vi "RestartPC ver2016 - Labview.vi"() -> ()   [LabVIEW 2016]
uses:
  System.Windows.Forms
  System.Drawing
panel:
  out "error out 3":errorcluster
  in  "error in (no error)":errorcluster
  out "error out":errorcluster
  out "standard output":string
  out "error out 2":errorcluster
  in  "stop":bool
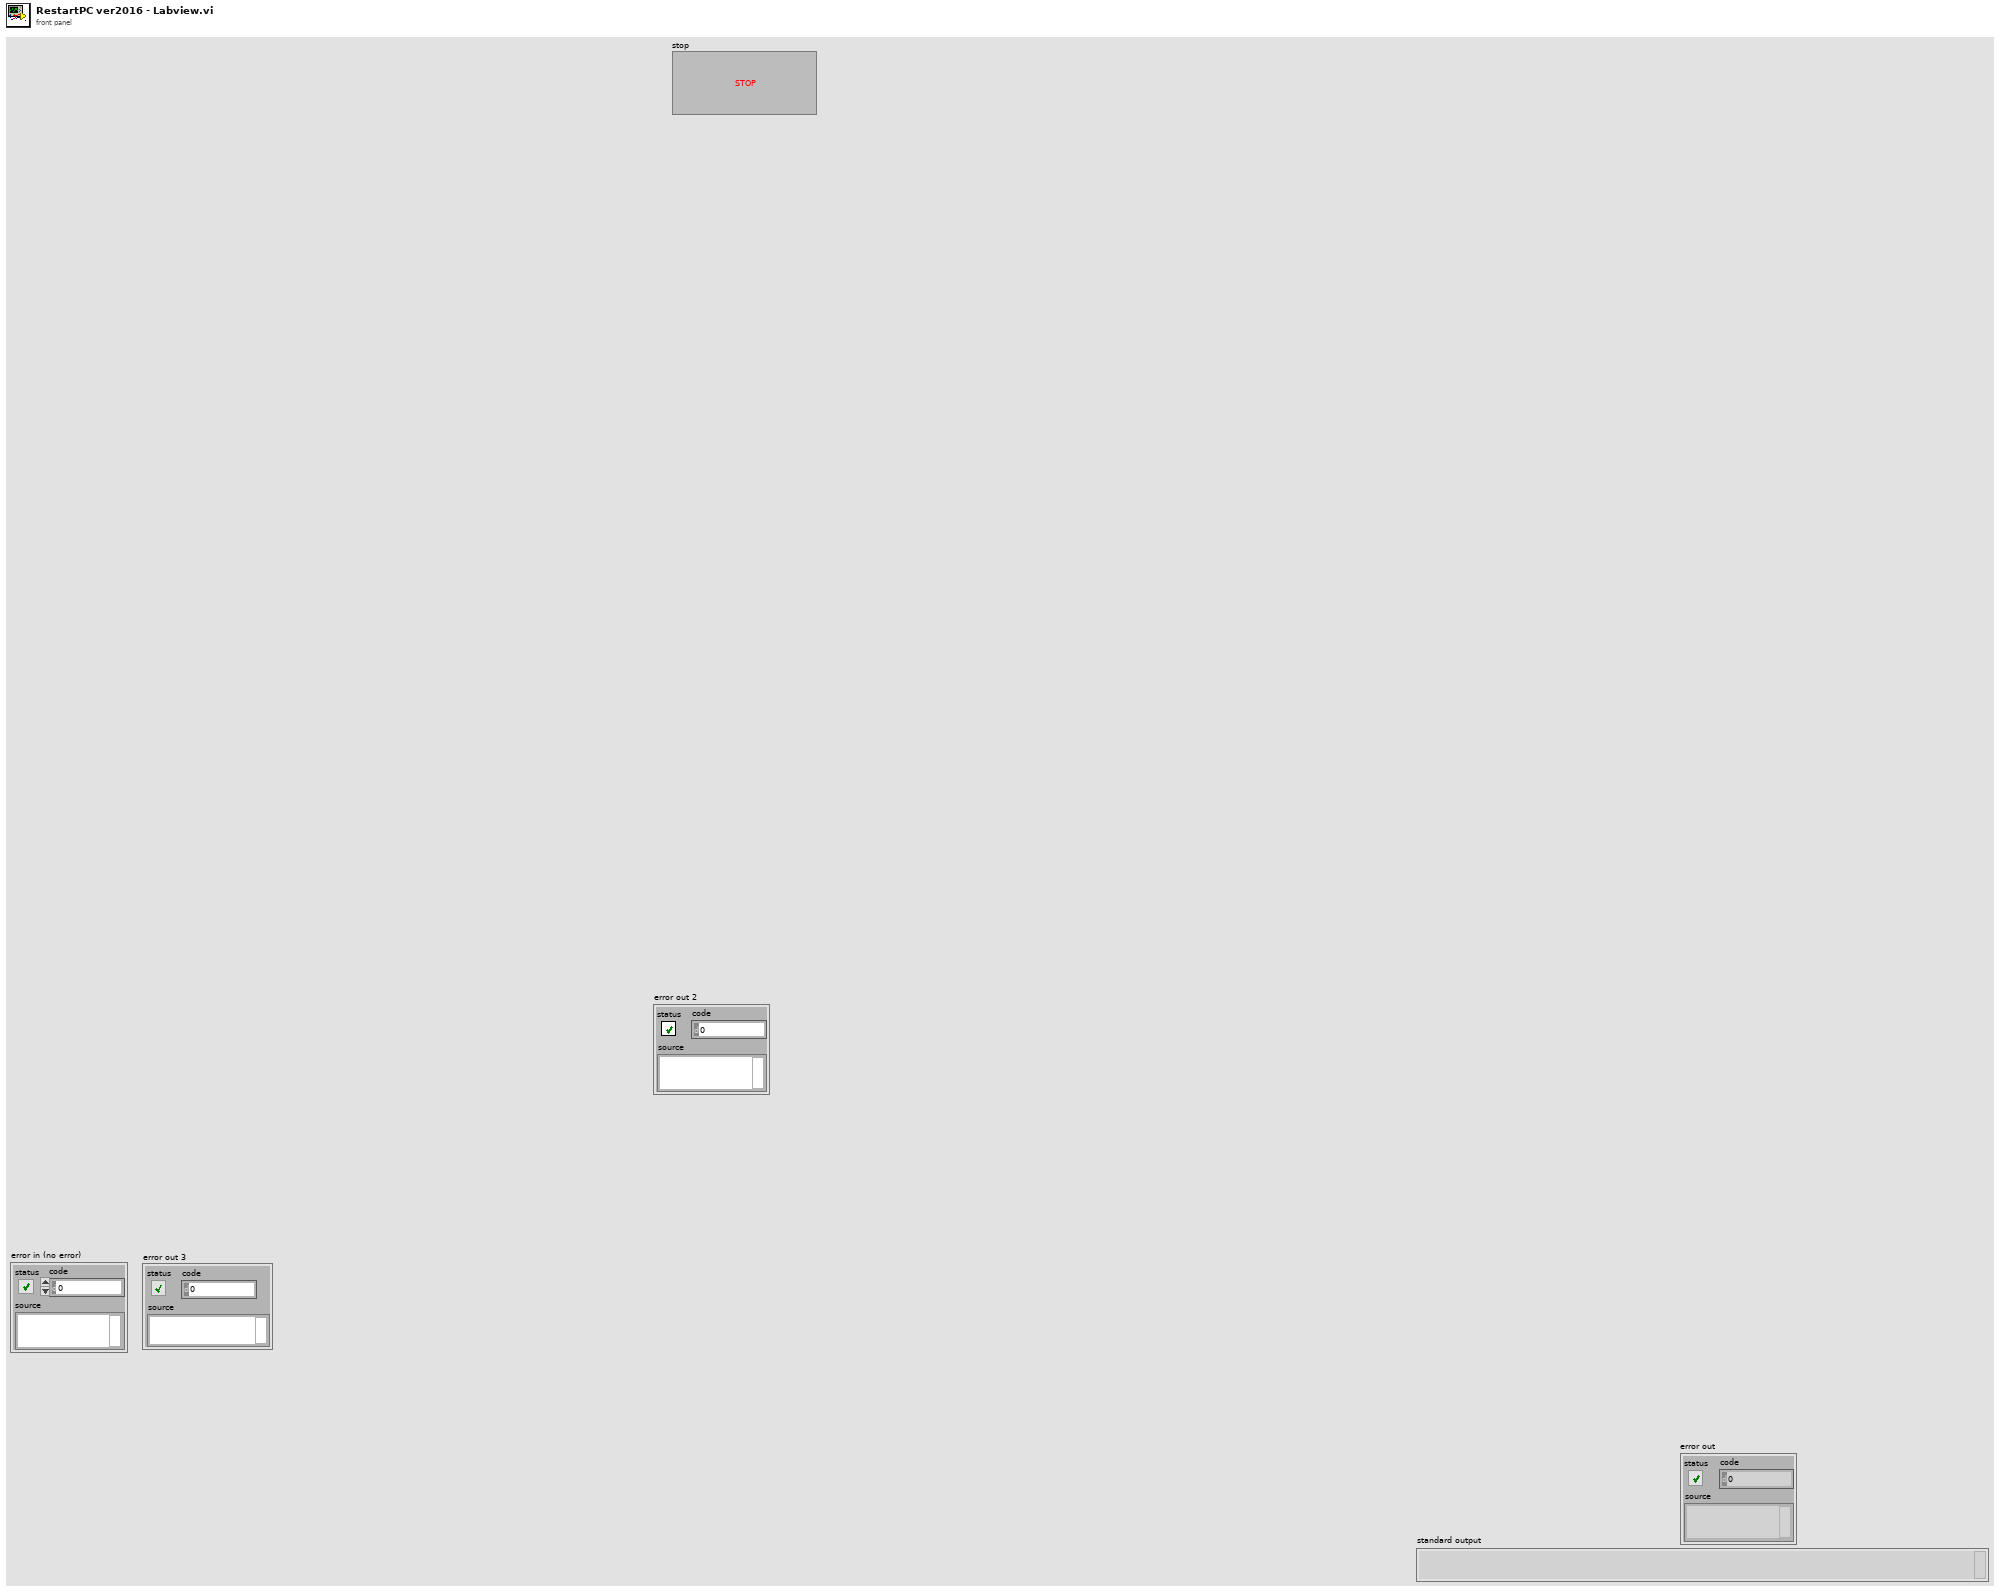
[diagram p1: front panel]
types:
  T1 = enum32{"Invalid", "Standard", "Closed", "Hidden", "Minimized", "Maximized"}
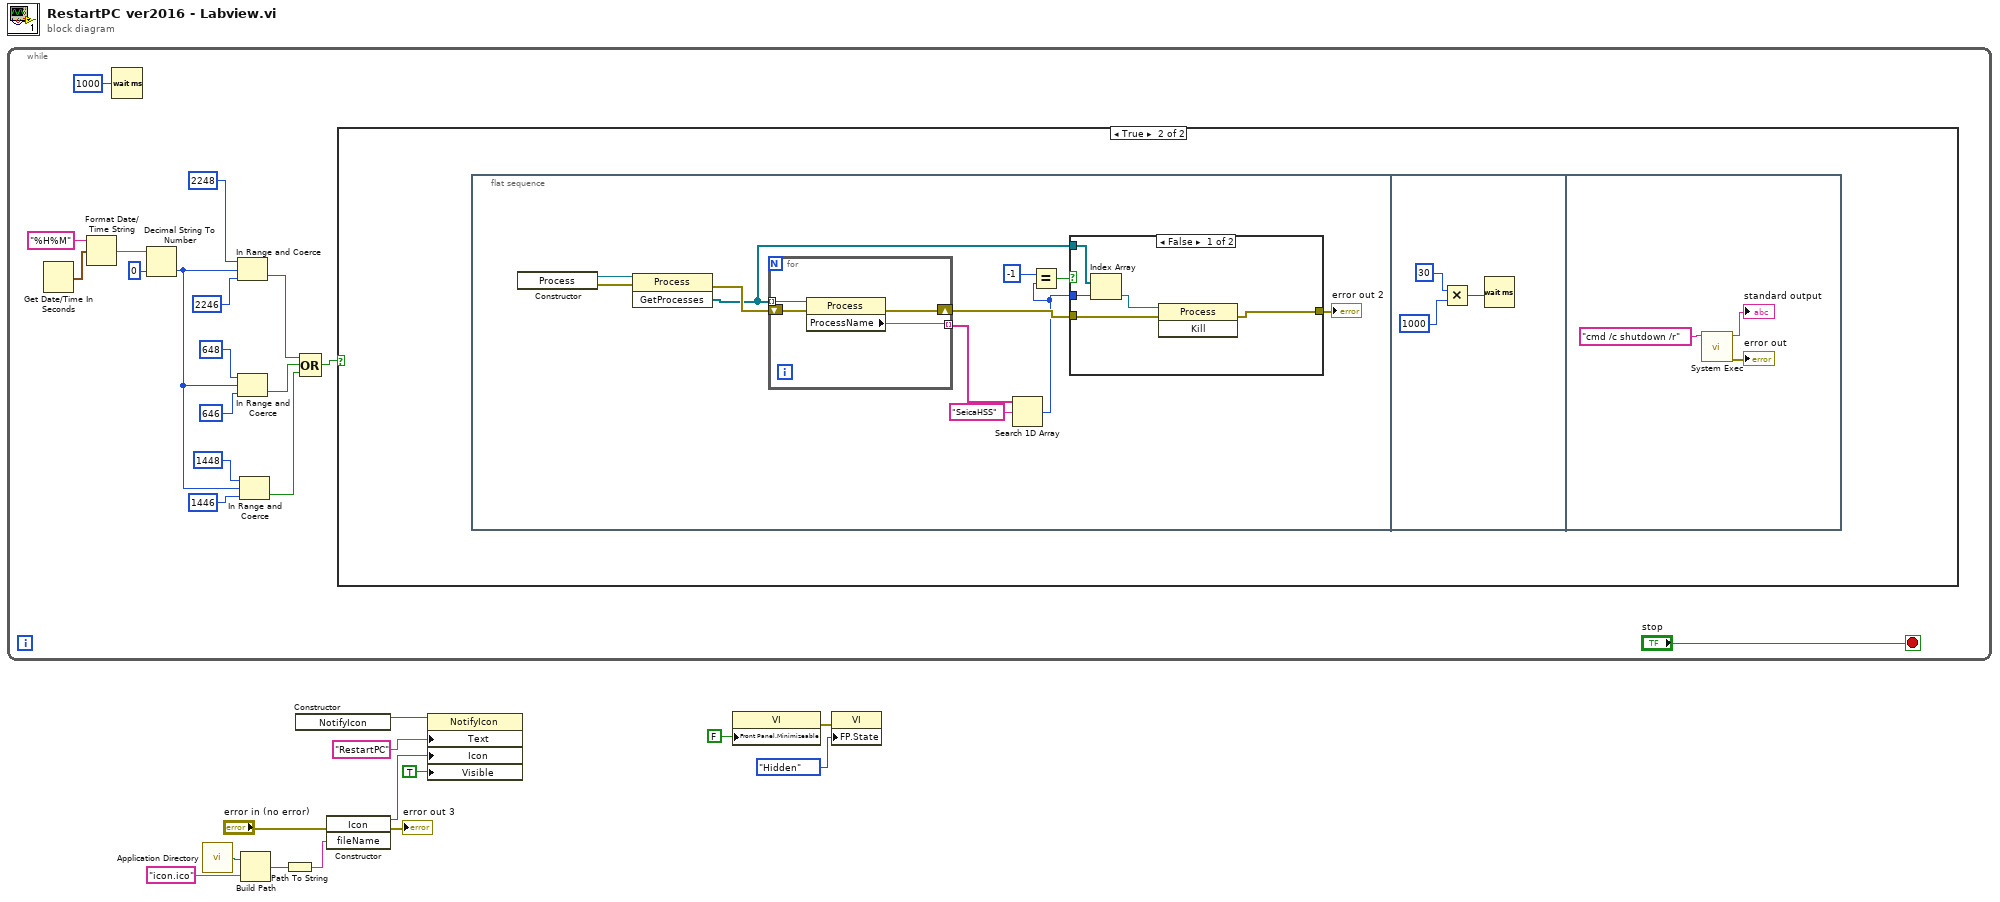
[diagram p0: block diagram]
diagram:
  n1 = while {
    stop <- "stop" stop-if-true
    n2 = Get Date/Time In Seconds() -> (seconds since 1Jan1904=w26:timestamp)
    n3 = Format Date/Time String(time format string (%c)="%H%M", seconds (now)=w26) -> (date/time string=w27:string)  [unwired: 1 in]
    n4 = Wait (ms)(milliseconds to wait=u32 1000) -> ()  [unwired: 1 out]
    n5 = Decimal String To Number(string=w27, default (0L)=0 ("default (0 I32)")) -> (number=w16:i32)  [unwired: 1 in, 1 out]
    n6 = In Range and Coerce(upper limit=2248, x=w16, lower limit=2246) -> (In Range?=w28:bool)  [unwired: 1 out]
    n7 = In Range and Coerce(upper limit=648, x=w16, lower limit=646) -> (In Range?=w29:bool)  [unwired: 1 out]
    n8 = In Range and Coerce(upper limit=1448, x=w16, lower limit=1446) -> (In Range?=w18:bool)  [unwired: 1 out]
    n9 = Compound Arithmetic op=OR(w28, w29, w18) -> (w30:bool)
    n10 = case shown="True" w30 {
      frame False {
      }
      frame True {
        n11 = flat-sequence {
          frame #0 {
            n12 = constructor class="Process"() -> (reference out=w41:refnum<k24>, error out=w40:errorcluster)  [unwired: 3 in, 1 out]
            n13 = invoke class="Process" method="GetProcesses"(reference=w41, error in=w40) -> (error out=w39:errorcluster, "GetProcesses"=w36:refnum<k24>[])  [unwired: 1 in, 1 out]
            n14 = for {
              tunnel: w36 -> [w51] mode=indexing
              shift-right: [w49] -> w35
              shift-left: w39 -> [w50]
              tunnel: [w48] -> w38 mode=indexing
              n15 = property class="Process"(reference=w51, error in=w50) -> (error out=w49:errorcluster, "ProcessName"=w48:string)  [unwired: 1 out]
            }
            n16 = Search 1D Array(1D array=w38, element="SeicaHSS") -> (index of element=w32:i32)  [unwired: 1 in]
            n17 = Equal?(x=-1, y=w32) -> (x = y?=w33:bool)
            n18 = case shown="False" w33 {
              tunnel: w32 -> [w46 _]
              tunnel: w36 -> [w45 _]
              tunnel: w35 -> [w43 w47]
              tunnel: [w42 w47] -> w34
              frame False {
                n19 = Index Array(array=w45, index=w46) -> (element=w44:refnum<k24>)
                n20 = invoke class="Process" method="Kill"(reference=w44, error in=w43) -> (error out=w42:errorcluster)  [unwired: 1 in, 2 out]
              }
              frame True {
              }
            }
            "error out 2" <- w34
          }
          frame #1 {
            n21 = Multiply(x=30, y=u32 1000 ("milliseconds to wait")) -> (x*y=w54:u32)
            n22 = Wait (ms)(milliseconds to wait=w54) -> ()  [unwired: 1 out]
          }
          frame #2 {
            n23 = call <vilib>:"System Exec.vi"("command line"="cmd /c shutdown /r") -> ("error out"=→"error out":errorcluster, "standard output"=→"standard output":string)  [unwired: 7 in, 2 out]
          }
        }
      }
    }
  }
  n24 = call <vilib>:"Application Directory.vi"() -> ("Application Directory"=w4:path)
  n25 = Build Path(base path=w4, name or relative path="icon.ico") -> (appended path=w9:path)
  n26 = Path To String(path=w9) -> (string=w8:string)
  n27 = constructor class="NotifyIcon"() -> (reference out=w13:refnum<k24>)  [unwired: 3 in, 2 out]
  n28 = constructor class="Icon"(error in="error in (no error)", "fileName"=w8) -> (reference out=w7:refnum<k24>, error out=→"error out 3":errorcluster)  [unwired: 2 in, 2 out]
  n29 = property class="NotifyIcon"(reference=w13, "Text"="RestartPC", "Icon"=w7, "Visible"=TRUE) -> ()  [unwired: 1 in, 2 out]
  n30 = property class="VI"("Front Panel.Minimizeable"=FALSE ("Front Panel Window:Minimizable")) -> (error out=w2:errorcluster)  [unwired: 2 in, 1 out]
  n31 = property class="VI"(error in=w2, "FP.State"=T1."Hidden" ("Front Panel Window:State")) -> ()  [unwired: 1 in, 2 out]
